vi "PressureControl - 3He.vi"(8 "error in (no error)":errorcluster, 11 "VISA resource name":refnum<visa-resource-name>) -> (0 "error out":errorcluster, 2 "3HePressure (Torr)":string, 3 "VISA resource name out":refnum<visa-resource-name>)   [LabVIEW 2018]
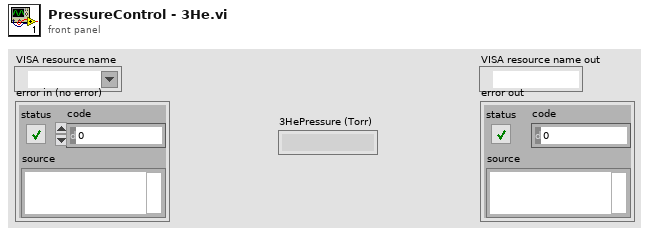
[diagram p1: front panel]
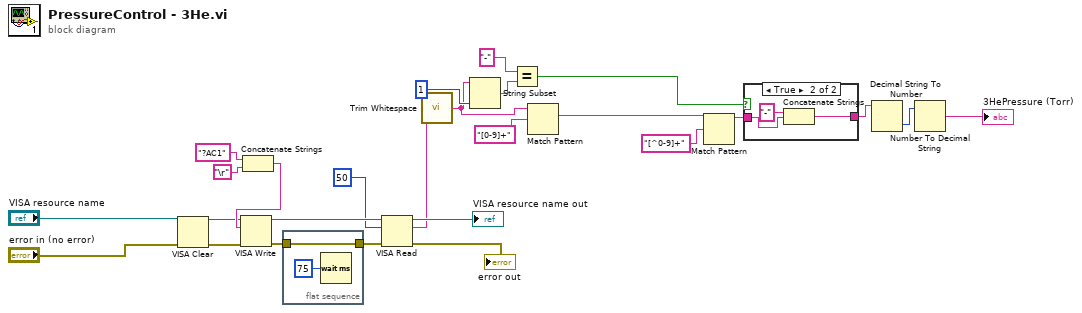
[diagram p0: block diagram]
diagram:
  n1 = VISA Clear(VISA resource name="VISA resource name", error in (no error)="error in (no error)") -> (VISA resource name out=w16:refnum<visa-resource-name>, error out=w17:errorcluster)
  n2 = Concatenate Strings("?AC1" ("write buffer"), "\r") -> (w18:string)
  n3 = VISA Write(VISA resource name=w16, write buffer=w18, error in (no error)=w17) -> (VISA resource name out=w25:refnum<visa-resource-name>, error out=w26:errorcluster)  [unwired: 1 out]
  n4 = flat-sequence {
    tunnel: w26 -> [w27]
    tunnel: [w27] -> w24
    frame #0 {
      n5 = Wait (ms)(milliseconds to wait=u32 75) -> ()  [unwired: 1 out]
    }
  }
  n6 = VISA Read(VISA resource name=w25, byte count=u32 50, error in (no error)=w24) -> (VISA resource name out=→"VISA resource name out":refnum<visa-resource-name>, read buffer=w14:string, error out=→"error out":errorcluster)  [unwired: 1 out]
  n7 = call "Trim Whitespace.vi"("string"=w14) -> ("trimmed string"=w9:string)  [unwired: 1 in]
  n8 = String Subset(string=w9, length (rest)=1 ("length (rest)")) -> (substring=w8:string)  [unwired: 1 in]
  n9 = Equal?(x="-", y=w8) -> (x = y?=w6:bool)
  n10 = Match Pattern(string=w9, regular expression="[0-9]+") -> (match substring=w4:string)  [unwired: 1 in, 3 out]
  n11 = Match Pattern(string=w4, regular expression="[^0-9]+") -> (before substring=w5:string)  [unwired: 1 in, 3 out]
  n12 = case shown="True" w6 {
    tunnel: w5 -> [w29 w31]
    tunnel: [w29 w30] -> w3
    frame False {
    }
    frame True {
      n13 = Concatenate Strings("-" ("string"), w31) -> (w30:string)
    }
  }
  n14 = Decimal String To Number(string=w3) -> (number=w2:i32)  [unwired: 2 in, 1 out]
  n15 = Number To Decimal String(number=w2) -> (decimal integer string=→"3HePressure (Torr)":string)  [unwired: 1 in]
